vi "Wait Until Generation Complete.vi"(8 "error in":errorcluster, 9 "duration":dbl, 10 "measurement context in":refnum<class "Measure Call Context.lvclass">, 11 "instrument handle in":refnum<k15>) -> (0 "error out":errorcluster, 1 "actual duration":dbl, 2 "measurement context out":refnum<class "Measure Call Context.lvclass">, 3 "instrument handle out":refnum<k15>)   [LabVIEW 2024, in "NIFgenSignalVoltageGeneration.lvlib"]
uses:
  <vilib>/MeasurementLink/MeasurementLink Measurement Server/Measure Call Context/Measure Call Context.lvclass
  <vilib>/MeasurementLink/MeasurementLink Measurement Server/Measure Call Context/Accessor/Is Canceled.vi
  NIFgenSignalVoltageGeneration.lvlib
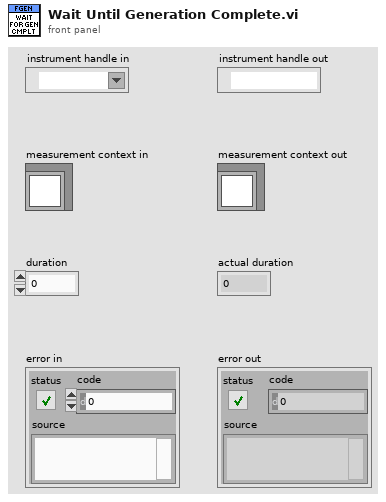
[diagram p1: front panel]
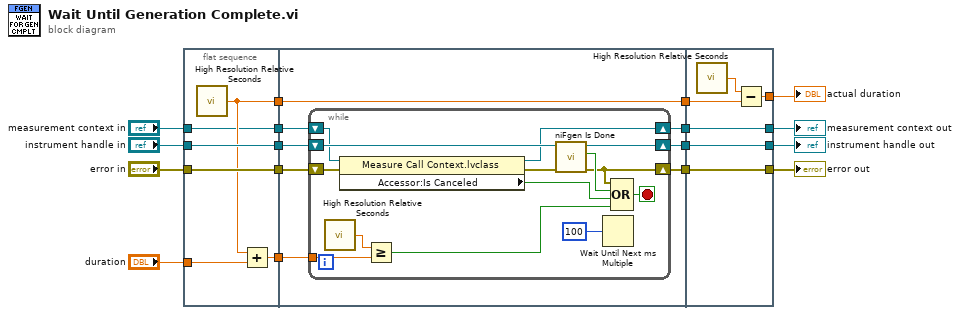
[diagram p0: block diagram]
diagram:
  n1 = flat-sequence {
    tunnel: "duration" -> [w21]
    tunnel: "instrument handle in" -> [w22]
    tunnel: "error in" -> [w23]
    tunnel: [w23] -> w17
    tunnel: [w22] -> w16
    tunnel: [w20] -> w15
    tunnel: [w19] -> w14
    tunnel: [w18] -> w13
    tunnel: "measurement context in" -> [w18]
    tunnel: w17 -> [w29]
    tunnel: w16 -> [w30]
    tunnel: w15 -> [w31]
    tunnel: [w28] -> w12
    tunnel: [w27] -> w11
    tunnel: [w31] -> w10
    tunnel: w14 -> [w26]
    tunnel: w13 -> [w25]
    tunnel: [w24] -> w9
    tunnel: [w50] -> w5
    tunnel: [w51] -> w4
    tunnel: w12 -> [w51]
    tunnel: w11 -> [w50]
    tunnel: w10 -> [w49]
    tunnel: [w48] -> w6
    tunnel: [w46] -> w8
    tunnel: w9 -> [w46]
    frame #0 {
      n2 = call <vilib>:"High Resolution Relative Seconds.vi"() -> ("relative seconds"=w20:dbl)
      n3 = Add(x=w20, y=w21) -> (x+y=w19:dbl)
    }
    frame #1 {
      n4 = while {
        shift-right: [w41] -> w27
        shift-left: w30 -> [w42]
        shift-right: [w34] -> w28
        shift-left: w29 -> [w36]
        tunnel: w26 -> [w45]
        shift-right: [w37] -> w24
        shift-left: w25 -> [w38]
        stop <- w39 stop-if-true
        n5 = call <vilib>:"High Resolution Relative Seconds.vi"() -> ("relative seconds"=w44:dbl)
        n6 = property class="Measure Call Context.lvclass"(reference=w38, error in=w36) -> (reference out=w37:refnum<class "Measure Call Context.lvclass">, error out=w35:errorcluster, "Accessor:Is Canceled"=w33:bool)
        n7 = Greater Or Equal?(x=w44, y=w45) -> (x >= y?=w32:bool)
        n8 = call <instrlib>:"niFgen Is Done.vi"("error in (no error)"=w35, "Instrument Handle"=w42) -> ("error out"=w34:errorcluster, "Done"=w40:bool, "Instrument Handle Out"=w41:refnum<k15>)  [unwired: 7 in]
        n9 = Wait Until Next ms Multiple(millisecond multiple=u32 100) -> ()  [unwired: 1 out]
        n10 = Compound Arithmetic op=OR(w34, w40, w33, w32) -> (w39:bool)
      }
    }
    frame #2 {
      n11 = call <vilib>:"High Resolution Relative Seconds.vi"() -> ("relative seconds"=w47:dbl)
      n12 = Subtract(x=w47, y=w49) -> (x-y=w48:dbl)
    }
  }
  "measurement context out" <- w8
  "actual duration" <- w6
  "instrument handle out" <- w5
  "error out" <- w4
